vi "_check_B.vi"(1 "输入":i8[](array[numeric]), 2 "n":dbl=3.0) -> (0 "输出":i8[](array[numeric]))   [LabVIEW 2018]
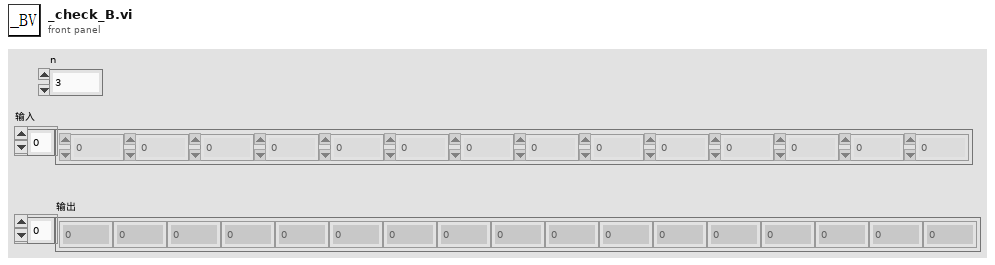
[diagram p1: front panel]
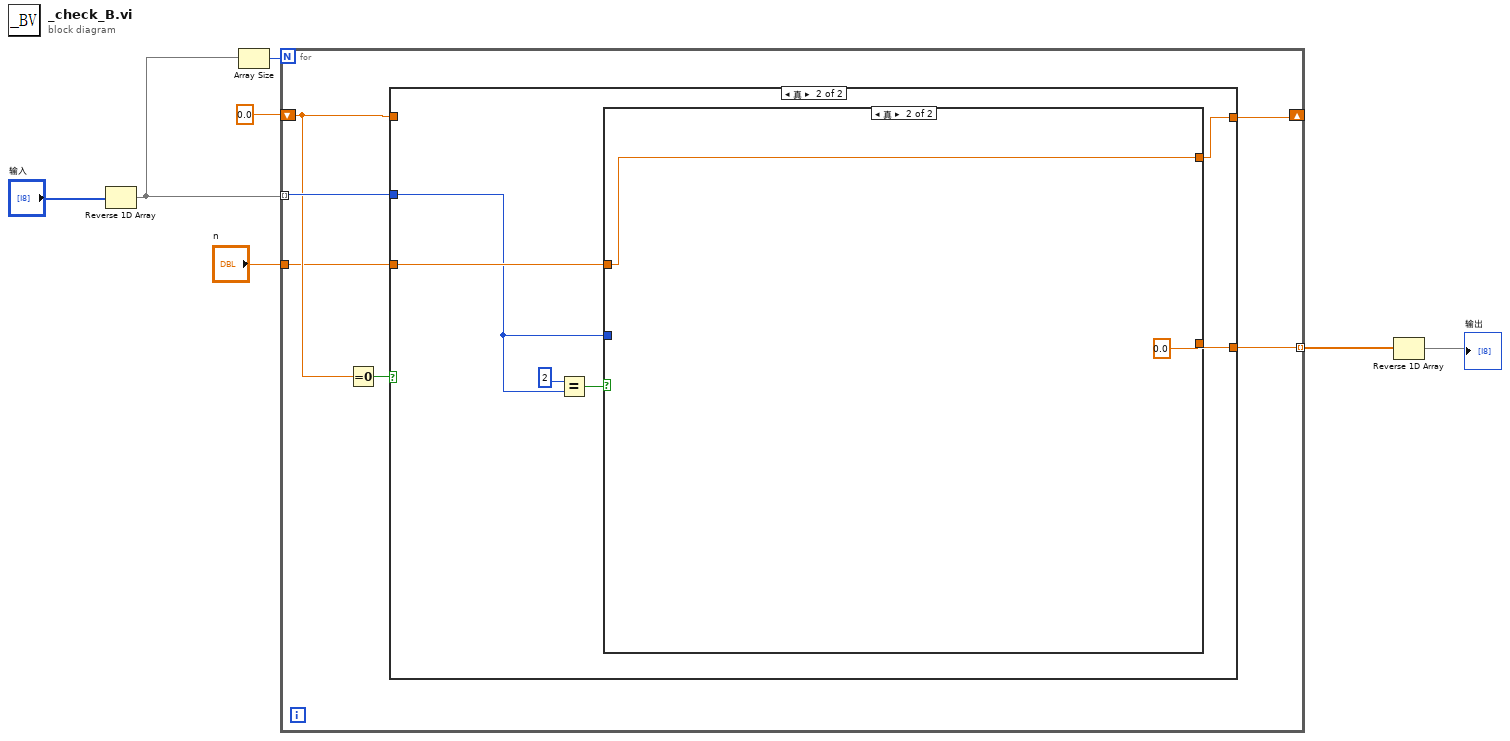
[diagram p0: block diagram]
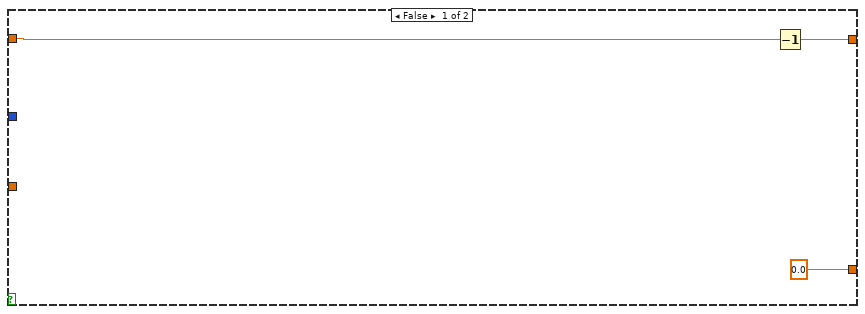
[diagram p2: hidden frame]
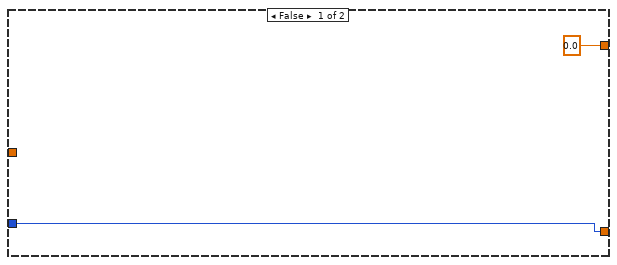
[diagram p3: hidden frame]
diagram:
  n1 = Reverse 1D Array(array="输入") -> (reversed array=w4:i8[])
  n2 = Array Size(array=w4) -> (size(s)=w5:i32)
  n3 = for {
    N: w5 -> [_]
    tunnel: w4 -> [w13] mode=indexing
    shift-right: [w10] -> _
    shift-left: 0.0 -> [w11]
    tunnel: [w9] -> w2 mode=indexing
    tunnel: "n" -> [w8]
    n4 = Equal To 0?(x=w11) -> (x = 0?=w12:bool)
    n5 = case shown="真" w12 {
      tunnel: w13 -> [_ w17]
      tunnel: w11 -> [w16 _]
      tunnel: [w15 w18] -> w10
      tunnel: [0.0 w20] -> w9
      tunnel: w8 -> [_ w19]
      frame False {
        n6 = Decrement(x=w16) -> (x-1=w15:dbl)
      }
      frame True {
        n7 = Equal?(x=i8 2, y=w17) -> (x = y?=w21:bool)
        n8 = case shown="真" w21 {
          tunnel: [w24 0.0] -> w20
          tunnel: w19 -> [_ w25]
          tunnel: [0.0 w25] -> w18
          tunnel: w17 -> [w24 _]
          frame False {
          }
          frame True {
          }
        }
      }
    }
  }
  n9 = Reverse 1D Array(array=w2) -> (reversed array=→"输出":dbl[])
